vi "KProp-Split Arg List.vi"(0 "Args":string[](array[string])) -> (4 "Properties":string[](array[string]), 8 "Values":string[](array[string]))   [LabVIEW 2020, in "KPropertyTable.xctl"]
uses:
  KPropertyTable.xctl
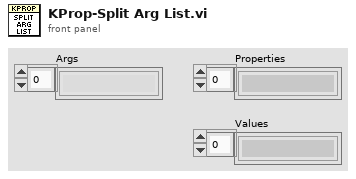
[diagram p1: front panel]
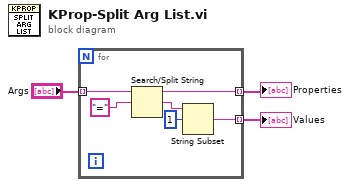
[diagram p0: block diagram]
diagram:
  n1 = for {
    tunnel: "Args" -> [w9] mode=indexing
    tunnel: [w7] -> w2 mode=indexing
    tunnel: [w4] -> w1 mode=indexing
    n2 = Search/Split String(string=w9, search string/char (-)="=") -> (substring before match=w7:string, match + rest of string=w6:string)  [unwired: 1 in, 1 out]
    n3 = String Subset(string=w6, offset (0)=1) -> (substring=w4:string)  [unwired: 1 in]
  }
  "Values" <- w1
  "Properties" <- w2
